vi "Cleanup.vi"(8 "error in (no error)":errorcluster, 11 "Group Buffer DBL in":refnum<class "Group Buffer DBL.lvclass">) -> (0 "error out":errorcluster)   [LabVIEW 2020, in "VolatusHistorian.lvlib" / "Group Buffer DBL.lvclass"]
uses:
  Group Buffer DBL.lvclass
  Group Buffer DBL.lvclass/Group Buffer DBL.ctl
  Channel Buffer DBL/Channel Buffer DBL.lvclass
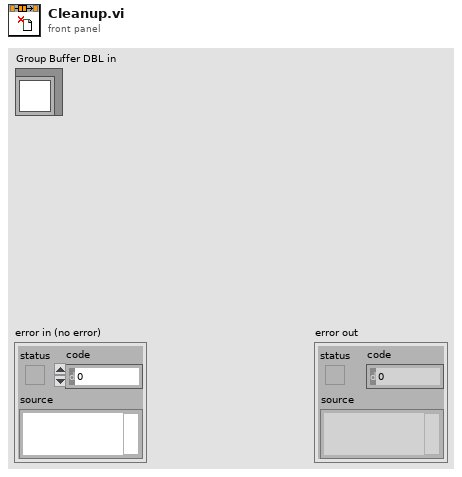
[diagram p1: front panel]
types:
  T1 = typedef "VolatusHistorian.lvlib/Group Buffer DBL.lvclass/Ref.ctl" = cluster{"Time":refnum<queue>, "Channel Name Map":map{string, i32}, "Group Info":T2, "Channels":refnum<class "Channel Buffer DBL.lvclass">[], "Channel Names":string[]}
  T2 = typedef "VectoConfig.lvlib/Group Info.ctl" = cluster{"System":string, "Cluster":string, "Node":string, "Task":string, "Name":string}
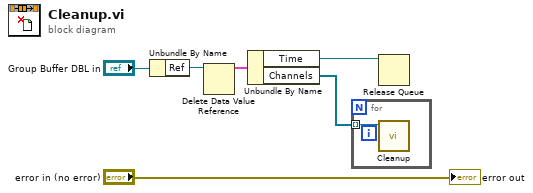
[diagram p0: block diagram]
diagram:
  n1 = Unbundle By Name("Group Buffer DBL in") -> ("Ref"=w4:refnum<data-value>)
  n2 = Delete Data Value Reference(data value reference=w4) -> (data value=w3:T1)  [unwired: 1 in, 1 out]
  n3 = Unbundle By Name(w3) -> ("Time"=w1:refnum<queue>, "Channels"=w2:refnum<class "Channel Buffer DBL.lvclass">[])
  n4 = for {
    tunnel: w2 -> [w7] mode=indexing
    n5 = call "Cleanup.vi"("Channel Buffer DBL in"=w7) -> ()  [unwired: 10 in, 1 out]
  }
  n6 = Release Queue(queue=w1) -> ()  [unwired: 2 in, 3 out]
  "error out" <- "error in (no error)"
